vi "p46_3_state.vi"() -> ()   [LabVIEW 2013]
uses:
  <vilib>/robotics/Kinematics/NI_Kinematics.lvlib
panel:
  out "state (x)":dbl[][](array[numeric])
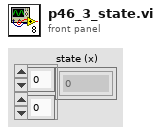
[diagram p1: front panel]
types:
  T1 = typedef "NI_Matrix.lvlib/RealMatrix.ctl" = dbl[][]
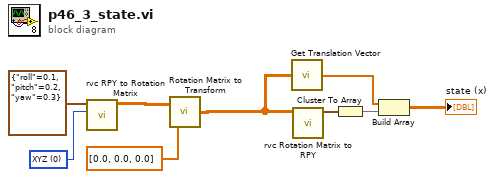
[diagram p0: block diagram]
diagram:
  w8 = u16 0 items=["XYZ", "ZYX"] ("Convension")
  n1 = call "rvc RPY to Rotation Matrix.vi"("Convension"=w8, "angles"=cluster{"roll":dbl, "pitch":dbl, "yaw":dbl} {"roll"=0.1, "pitch"=0.2, "yaw"=0.3}) -> ("rotation matrix"=w7:T1)  [unwired: 9 in]
  n2 = call <vilib>:"Rotation Matrix to Transform.vi"("translation vector"=dbl[] [0.0, 0.0, 0.0], "rotation matrix"=w7) -> ("transform"=w4:T1)
  n3 = call <vilib>:"Get Translation Vector.vi"("transform"=w4) -> ("translation vector"=w2:dbl[])
  n4 = call "rvc Rotation Matrix to RPY.vi"("rotation matrix"=w4) -> ("angles"=w5:cluster{"roll":dbl, "pitch":dbl, "yaw":dbl})  [unwired: 10 in]
  n5 = Cluster To Array(cluster=w5) -> (array=w3:dbl[])
  n6 = Build Array(w2, w3) -> (→"state (x)":dbl[][])
